vi "Creating Modulated Audio.vi"() -> ()   [LabVIEW 2019]
doc: "This application reads the selected audio file from its media storage. The audio is outputed through the Emona Communications Board for its modulation. After being modulated, the signal is inputed once again into the application. The modulated signal is now displayed through the Modulated Signal Graph."
uses:
  <vilib>/myRIO/Instrument Drivers/Onboard IO/AO Continuous/typedefs/AO Continuous Reference.ctl
  <vilib>/myRIO/Common/Instrument Driver Framework/Utilities/typedefs/myRIO Generic Hardware Reference.ctl
  <vilib>/myRIO/Common/Instrument Driver Framework/Utilities/typedefs/Hardware Version Enum.ctl
  <vilib>/myRIO/Common/Instrument Driver Framework/Utilities/typedefs/myRIO v1.0 Reference.ctl
  <vilib>/myRIO/Common/Instrument Driver Framework/Utilities/typedefs/Generic FPGA Reference.ctl
  <vilib>/myRIO/Common/Instrument Driver Framework/ELVIS III v1.0/AO Continuous/typedefs/AO Continuous Channels List.ctl
  <vilib>/myRIO/Common/Instrument Driver Framework/ELVIS III v1.0/AO Continuous/typedefs/ELVIS III v1.0 AO Continuous Channels Enum.ctl
  <vilib>/myRIO/Common/Instrument Driver Framework/ELVIS III v1.0/AO Continuous/typedefs/AO Continuous Channel Info.ctl
  <vilib>/userDefined/High Color/nirio_resource_hc.ctl
  <vilib>/myRIO/Instrument Drivers/Onboard IO/AO/typedefs/AO Reference.ctl
  <vilib>/myRIO/Common/Instrument Driver Framework/myRIO v1.0/AO/typedefs/AO Channels List.ctl
  <vilib>/myRIO/Common/Instrument Driver Framework/myRIO v1.0/AO/typedefs/AO Channels Enum.ctl
  <vilib>/myRIO/Common/Instrument Driver Framework/Utilities/typedefs/Analog Scaling Constants List.ctl
  <vilib>/myRIO/Common/Instrument Driver Framework/Utilities/typedefs/Analog Scaling Constants.ctl
  <vilib>/myRIO/Instrument Drivers/Onboard IO/AI Block/typedefs/AI Block Reference.ctl
  <vilib>/myRIO/Common/Instrument Driver Framework/myRIO v1.0/AI Block/typedefs/AI Block Channels List.ctl
  <vilib>/myRIO/Common/Instrument Driver Framework/myRIO v1.0/AI Block/typedefs/AI Block Channels Enum.ctl
  <vilib>/myRIO/Common/Instrument Driver Framework/ELVIS III v1.0/AO Continuous/vis/ELVIS III v1.1 Open AO (Continuous).vi
  <vilib>/myRIO/Common/Instrument Driver Framework/ELVIS III v1.0/AO/vis/ELVIS III v1.1 Open AO.vi
  <vilib>/myRIO/Common/Instrument Driver Framework/ELVIS III v1.0/AI Block/vis/ELVIS III v1.1 Open AI (N Samples).vi
  <vilib>/myRIO/Common/Instrument Driver Framework/Utilities/vis/Validate Channels.vi
  <vilib>/myRIO/Common/Instrument Driver Framework/ELVIS III v1.0/AO Continuous/vis/ELVIS III v1.0 Reserve AO Continuous.vi
  <vilib>/myRIO/Common/Instrument Driver Framework/ELVIS III v1.0/AO/vis/ELVIS III v1.0 Reserve AO.vi
  <vilib>/myRIO/Common/Instrument Driver Framework/ELVIS III v1.0/Resource Manager/vis/ELVIS III v1.0 Check For Different Banks.vi
  <vilib>/myRIO/Common/Instrument Driver Framework/ELVIS III v1.0/AI Block/vis/ELVIS III v1.0 AI Block Read.vi
  <vilib>/myRIO/Common/Instrument Driver Framework/ELVIS III v1.0/AO Continuous/vis/ELVIS III v1.1 Close AO Continuous.vi
  <vilib>/myRIO/Common/Instrument Driver Framework/ELVIS III v1.0/AO/vis/ELVIS III v1.0 Close AO.vi
  <vilib>/myRIO/Common/Instrument Driver Framework/ELVIS III v1.0/AI Block/vis/ELVIS III v1.0 Close AI Block.vi
  <vilib>/myRIO/Common/Instrument Driver Framework/myRIO v1.0/UART/vis/myRIO v1.0 Close UART.vi
  <vilib>/myRIO/Common/Instrument Driver Framework/ELVIS III v1.0/AO Continuous/vis/ELVIS III v1.0 Build MUX Configuration AO Continuous.vi
  <vilib>/myRIO/Common/Instrument Driver Framework/ELVIS III v1.0/AO/vis/ELVIS III v1.0 Build MUX Configuration AO.vi
  <vilib>/myRIO/Common/Instrument Driver Framework/Utilities/vis/Sample Rate To Ticks.vi
  <vilib>/myRIO/Common/Instrument Driver Framework/ELVIS III v1.0/AO Continuous/vis/ELVIS III v1.0 Unreserve AO Continuous.vi
  <vilib>/myRIO/Common/Instrument Driver Framework/ELVIS III v1.0/AO/vis/ELVIS III v1.0 Unreserve AO.vi
  <vilib>/myRIO/Common/Instrument Driver Framework/ELVIS III v1.0/AI Block/vis/ELVIS III v1.0 Unreserve AI Block.vi
  <vilib>/myRIO/Common/Instrument Driver Framework/ELVIS III v1.0/AI Block/vis/ELVIS III v1.0 Build MUX Configuration AI Block.vi
  <vilib>/Utility/VariantDataType/GetNumericInfo.vi
  <vilib>/Utility/error.llb/Error Cluster From Error Code.vi
  <vilib>/myRIO/Common/Instrument Driver Framework/ELVIS III v1.0/ELVIS III v1.1 Open.vi
  <vilib>/myRIO/Common/Instrument Driver Framework/ELVIS III v1.0/Resource Manager/vis/ELVIS III v1.0 Coerce AI Scaling.vi
  <vilib>/myRIO/Common/Instrument Driver Framework/ELVIS III v1.0/AI Block/vis/ELVIS III v1.0 Reserve AI Block.vi
  <vilib>/myRIO/Common/Instrument Driver Framework/ELVIS III v1.0/Resource Manager/vis/ELVIS III v1.0 Configure DMAs.vi
  <vilib>/myRIO/Common/Instrument Driver Framework/myRIO v1.0/myRIO v1.0 Close.vi
  <vilib>/myRIO/Common/Instrument Driver Framework/ELVIS III v1.0/Resource Manager/vis/ELVIS III v1.0 Reserve Channel List.vi
  <vilib>/myRIO/Common/Instrument Driver Framework/ELVIS III v1.0/AO Continuous/vis/ELVIS III v1.1 Stop AO Continuous.vi
  <vilib>/myRIO/Common/Instrument Driver Framework/ELVIS III v1.0/AO Continuous/vis/ELVIS III v1.0 AO Continuous Write.vi
  <vilib>/myRIO/Common/Instrument Driver Framework/ELVIS III v1.0/AO/vis/ELVIS III v1.0 Write AO.vi
  <vilib>/myRIO/Common/Instrument Driver Framework/ELVIS III v1.0/AO Continuous/vis/ELVIS III v1.1 Start AO Continuous.vi
  <vilib>/myRIO/Common/Instrument Driver Framework/myRIO v1.0/Resource Manager/vis/myRIO v1.0 Block Write Configuration.vi
  <vilib>/myRIO/Common/Instrument Driver Framework/ELVIS III v1.0/AI Block/vis/ELVIS III v1.0 AI Block Read Bank A.vi
  <vilib>/myRIO/Common/Instrument Driver Framework/ELVIS III v1.0/AI Block/vis/ELVIS III v1.0 AI Block Read Bank B.vi
  <vilib>/myRIO/Common/Instrument Driver Framework/ELVIS III v1.0/Resource Manager/vis/ELVIS III v1.0 Unreserve Channel List.vi
  <vilib>/myRIO/Common/Instrument Driver Framework/Utilities/vis/FPGA Ref Manager.vi
  <vilib>/myRIO/Common/Instrument Driver Framework/ELVIS III v1.0/ELVIS III v1.0 Reset FPGA.vi
  <vilib>/myRIO/Common/Instrument Driver Framework/myRIO v1.0/IRQ/vis/myRIO v1.0 IRQ Info FGV.vi
  <vilib>/myRIO/Common/Instrument Driver Framework/myRIO v1.0/IRQ/vis/myRIO v1.0 Timer IRQ Info FGV.vi
  <vilib>/myRIO/Common/Instrument Driver Framework/myRIO v1.0/IRQ/vis/myRIO v1.0 ISR Agent.vi
  <vilib>/myRIO/Instrument Drivers/Utilities/vis/Reset Index.vi
  <vilib>/myRIO/Common/Instrument Driver Framework/myRIO v1.0/Resource Manager/vis/myRIO v1.0 Block Write Resource Manager.vi
  <vilib>/myRIO/Instrument Drivers/Onboard IO/AI Block/vis/myRIO AI N Samples Open.xnode
  <vilib>/myRIO/Instrument Drivers/Onboard IO/AO/vis/myRIO AO Open.xnode
  <vilib>/myRIO/Instrument Drivers/Onboard IO/AO Continuous/vis/myRIO AO Continuous Open.xnode
  <vilib>/myRIO/Instrument Drivers/Utilities/Utilities.lvlib
  <vilib>/myRIO/Instrument Drivers/Onboard IO/AI Block/AI Block.lvlib
  <vilib>/myRIO/Instrument Drivers/Onboard IO/AO/AO.lvlib
  <vilib>/myRIO/Instrument Drivers/Onboard IO/AO Continuous/AO Continuous.lvlib
panel:
  in  "Select Audio":u16(ring)
  out "Message":dbl[](graph) caption="Message History"
  in  "Offset":dbl=1.0
  out "Modulated Signal":dbl[](graph)
  out "error out":errorcluster
  in  "Stop":bool
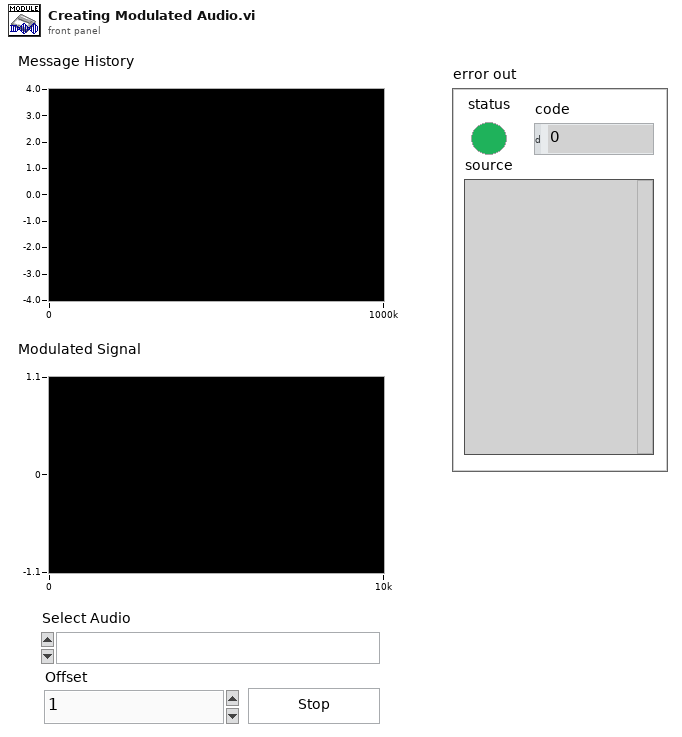
[diagram p1: front panel]
types:
  T1 = enum16{"open", "replace", "create", "open or create", "replace or create", "replace or create with confirmation"}
  T2 = typedef "nirio_resource_hc.ctl" = tag
  T3 = typedef "Hardware Version Enum.ctl" = enum16{"Unknown", "myRIO-1900", "myRIO-1950", "roboRIO", "NI ELVIS RIO CM", "ELVIS III"}
  T4 = typedef "AO Continuous.lvlib/AO Continuous Reference.ctl" = cluster{"myRIO Reference":T5, "AO (Continuous) Channels List":T8, "Channel Info":T10}
  T5 = typedef "myRIO Generic Hardware Reference.ctl" = cluster{"myRIO Model":T3, "myRIO Hardware Reference":T6}
  T6 = typedef "myRIO v1.0 Reference.ctl" = cluster{"Generic FPGA Reference":T7, "Allow multiple opens":bool}
  T7 = typedef "Generic FPGA Reference.ctl" = refnum<k20>
  T8 = typedef "AO Continuous Channels List.ctl" = T9[]
  T9 = typedef "ELVIS III v1.0 AO Continuous Channels Enum.ctl" = enum16{"Not Connected", "A/AO0 (Continuous)", "A/AO1 (Continuous)", "B/AO0 (Continuous)", "B/AO1 (Continuous)"}
  T10 = typedef "AO Continuous Channel Info.ctl" = cluster{"Channel Bitmask":u8[], "Channel Index":i32[], "Channel Number":u8}
  T11 = typedef "AO.lvlib/AO Reference.ctl" = cluster{"myRIO Reference":T5, "AO Channel List":T12, "AO Scaling Constant List":T14}
  T12 = typedef "AO Channels List.ctl" = T13[]
  T13 = typedef "AO Channels Enum.ctl" = enum16{"Not Connected", "AudioOut/Left", "AudioOut/Right", "C/AO0", "C/AO1", "A/AO0", "A/AO1", "B/AO0", "B/AO1"}
  T14 = typedef "Analog Scaling Constants List.ctl" = T15[]
  T15 = typedef "Analog Scaling Constants.ctl" = cluster{"LSB Weight (Volts)":dbl, "Offset (Volts)":dbl, "Signed?":bool}
  T16 = typedef "AI Block.lvlib/AI Block Reference.ctl" = cluster{"myRIO Reference":T5, "AI (N Samples) Channels List":T17, "AI (N Samples) Scaling Constants List":T15[]}
  T17 = typedef "AI Block Channels List.ctl" = T18[]
  T18 = typedef "AI Block Channels Enum.ctl" = enum16{"Not Connected", "A/AI0 (N Samples)", "A/AI1 (N Samples)", "A/AI2 (N Samples)", "A/AI3 (N Samples)", "A/AI4 (N Samples)", "A/AI5 (N Samples)", "A/AI6 (N Samples)", "A/AI7 (N Samples)", "A/AI0 (DIFF N Samples)", "A/AI1 (DIFF N Samples)", "A/AI2 (DIFF N Samples)", "A/AI3 (DIFF N Samples)", "B/AI0 (N Samples)", "B/AI1 (N Samples)", "B/AI2 (N Samples)", "B/AI3 (N Samples)", "B/AI4 (N Samples)", "B/AI5 (N Samples)", "B/AI6 (N Samples)", "B/AI7 (N Samples)", "B/AI0 (DIFF N Samples)", "B/AI1 (DIFF N Samples)", "B/AI2 (DIFF N Samples)", "B/AI3 (DIFF N Samples)"}
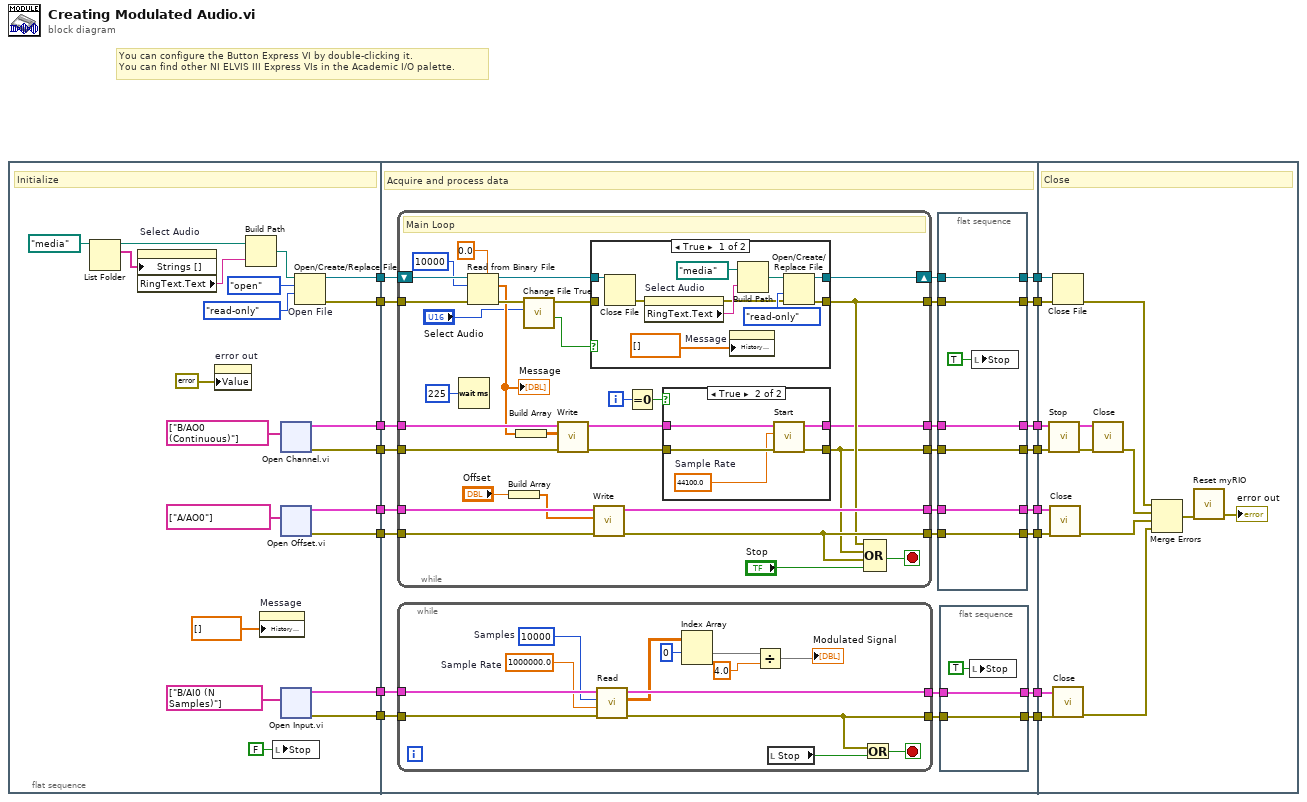
[diagram p0: block diagram]
diagram:
  # "You can configure the Button Express VI by double-clicking it.\nYou can find other NI ELVIS III Express VIs in the Academic I/O palette."
  n1 = flat-sequence {
    tunnel: [w36] -> w16
    tunnel: [w35] -> w15
    tunnel: [w33] -> w12
    tunnel: [w32] -> w11
    tunnel: [w27] -> w8
    tunnel: [w26] -> w7
    tunnel: [w23] -> w5
    tunnel: [w22] -> w4
    tunnel: w16 -> [w116]
    tunnel: w15 -> [w115]
    tunnel: [w93] -> w14
    tunnel: [w95] -> w13
    tunnel: w12 -> [w114]
    tunnel: w11 -> [w113]
    tunnel: [w99] -> w10
    tunnel: [w97] -> w9
    tunnel: w8 -> [w112]
    tunnel: w7 -> [w111]
    tunnel: [w105] -> w6
    tunnel: w5 -> [w110]
    tunnel: w4 -> [w109]
    tunnel: [w103] -> w3
    tunnel: [w101] -> w2
    tunnel: [w108] -> w1
    tunnel: w14 -> [w204]
    tunnel: w13 -> [w203]
    tunnel: w10 -> [w199]
    tunnel: w9 -> [w198]
    tunnel: w6 -> [w195]
    tunnel: w3 -> [w191]
    tunnel: w2 -> [w190]
    tunnel: w1 -> [w196]
    frame #0 {
      # "Initialize"
      n2 = List Folder(path=path "/media") -> (path out=w19:path, filenames=w20:string[])  [unwired: 3 in, 2 out]
      n3 = property on="Select Audio" class="Ring (strict)"("Strings []"=w20) -> ("RingText.Text"=w18:string)  [unwired: 2 in, 2 out]
      n4 = property on="error out" class="Clust (strict)"("Value"=errorcluster {"status"=FALSE, "code"=0, "source"=""} ("error constant")) -> ()  [unwired: 2 in, 2 out]
      n5 = Build Path(base path=w19, name or relative path=w18) -> (appended path=w28:path)
      n6 = property on="Message" class="WFChart (strict)"("History Data"=dbl[] []) -> ()  [unwired: 2 in, 2 out]
      n7 = local write "Stop"(FALSE ("Stop")) -> ()
      n8 = xnode "Open Channel.vi"("Channel Names"=tag[] ["B/AO0 (Continuous)"]) -> ("error out"=w22:errorcluster, "AO (Continuous) Ref Out"=w23:T4)  [unwired: 1 in]
      n9 = xnode "Open Offset.vi"("Channel Names"=tag[] ["A/AO0"]) -> ("error out"=w32:errorcluster, "AO Ref Out"=w33:T11)  [unwired: 2 in]
      n10 = xnode "Open Input.vi"("Channel Names"=tag[] ["B/AI0 (N Samples)"]) -> ("error out"=w36:errorcluster, "AI (N Samples) Ref Out"=w35:T16)  [unwired: 4 in]
      n11 = Open/Create/Replace File "Open File"(file path (use dialog)=w28, operation (0:open)=T1."open", access (0:read/write)=enum16{"read/write", "read-only", "write-only"}."read-only") -> (refnum out=w27:refnum<file>, error out=w26:errorcluster)  [unwired: 3 in, 1 out]
    }
    frame #1 {
      # "Acquire and process data"
      n12 = while {
        tunnel: w114 -> [w169]
        tunnel: w113 -> [w168]
        tunnel: [w165] -> w100
        tunnel: [w164] -> w98
        tunnel: w111 -> [w162]
        tunnel: [w155] -> w106
        tunnel: w109 -> [w149]
        tunnel: [w147] -> w102
        tunnel: w110 -> [w150]
        tunnel: [w148] -> w104
        shift-right: [w158] -> w107
        shift-left: w112 -> [w163]
        i -> [w151]
        stop <- w166 stop-if-true
        # "Main Loop"
        n13 = Wait (ms)(milliseconds to wait=u32 225) -> ()  [unwired: 1 out]
        n14 = Read from Binary File(5:0.0, 8:w162, 10:10000, 11:w163) -> (0:w145:errorcluster, 2:w142:dbl[], 3:w159:refnum<file>)  [unwired: 2 in, 1 out]
        "Message" <- w142
        n15 = Build Array("Offset") -> (w160:dbl[])
        n16 = Build Array(w142) -> (w146:dbl[][])
        n17 = call "Change File True.vi"("error in"=w145, "Numeric in"="Select Audio") -> ("error out"=w144:errorcluster, "Change song?"=w141:bool)  [unwired: 6 in, 1 out]
        n18 = call <vilib>:"Write.vi"("error in (no error)"=w149, "Data To Write"=w146, "AO (Continuous) Ref In"=w150) -> ("error out"=w153:errorcluster, "AO (Continuous) Ref Out"=w154:T4)  [unwired: 7 in]
        n19 = case shown="True" w141 {
          tunnel: [w183 w187] -> w155
          tunnel: w159 -> [w185 w188]
          tunnel: [w184 w188] -> w158
          tunnel: w144 -> [_ w187]
          frame True {
            n20 = Close File(refnum=w185) -> (error out=w178:errorcluster)  [unwired: 1 in, 1 out]
            n21 = property on="Select Audio" class="Ring (strict)"(error in=w178) -> (error out=w177:errorcluster, "RingText.Text"=w179:string)  [unwired: 1 in, 1 out]
            n22 = property on="Message" class="WFChart (strict)"("History Data"=dbl[] []) -> ()  [unwired: 2 in, 2 out]
            n23 = Build Path(base path=path "/media" ("path"), name or relative path=w179) -> (appended path=w181:path)
            n24 = Open/Create/Replace File ("Open File")(file path (use dialog)=w181, error in=w177, access (0:read/write)=enum16{"read/write", "read-only", "write-only"}."read-only") -> (refnum out=w184:refnum<file>, error out=w183:errorcluster)  [unwired: 3 in, 1 out]
          }
          frame False {
          }
        }
        n25 = call <vilib>:"Write.vi"("error in (no error)"=w168, "Values"=w160, "AO Ref In"=w169) -> ("error out"=w164:errorcluster, "AO Ref Out"=w165:T11)  [unwired: 6 in]
        n26 = Equal To 0?(x=w151) -> (x = 0?=w152:bool)
        n27 = case shown="True" w152 {
          tunnel: w154 -> [w171 w176]
          tunnel: w153 -> [w170 w175]
          tunnel: [w171 w174] -> w148
          tunnel: [w170 w173] -> w147
          frame False {
          }
          frame True {
            w172 = 44100.0  # Sample Rate
            n28 = call <vilib>:"Start.vi"("error in (no error)"=w175, "Sample Rate"=w172, "AO (Continuous) Ref In"=w176) -> ("error out"=w173:errorcluster, "AO (Continuous) Ref Out"=w174:T4)  [unwired: 7 in]
          }
        }
        n29 = Compound Arithmetic op=OR(w155, w147, w164, "Stop") -> (w166:bool)
      }
      n30 = while {
        tunnel: w115 -> [w139]
        tunnel: [w134] -> w96
        tunnel: w116 -> [w138]
        tunnel: [w136] -> w94
        stop <- w137 stop-if-true
        w128 = u32 10000  # Samples
        w129 = 1000000.0  # Sample Rate
        n31 = call <vilib>:"Read.vi"("error in (no error)"=w138, "Sample Rate [Hz]"=w129, "Number of Samples"=w128, "AI (N Samples) Ref In"=w139) -> ("error out"=w136:errorcluster, "Values"=w133:dbl[][], "AI (N Samples) Ref Out"=w134:T16)  [unwired: 5 in]
        n32 = Index Array(array=w133, index (row)=0) -> (element=w131:dbl[])  [unwired: 1 in]
        n33 = Divide(x=w131, y=4.0) -> (x/y=→"Modulated Signal":dbl[])
        n34 = local read "Stop"() -> (w135:bool)
        n35 = Or(x=w136, y=w135) -> (x .or. y?=w137:bool)
      }
      n36 = flat-sequence {
        tunnel: [w126] -> w108
        tunnel: w107 -> [w126]
        tunnel: w106 -> [w125]
        tunnel: [w125] -> w105
        tunnel: w104 -> [w124]
        tunnel: [w124] -> w103
        tunnel: w102 -> [w123]
        tunnel: [w123] -> w101
        tunnel: w100 -> [w122]
        tunnel: [w122] -> w99
        tunnel: w98 -> [w121]
        tunnel: [w121] -> w97
        frame #0 {
          n37 = local write "Stop"(TRUE ("Stop")) -> ()
        }
      }
      n38 = flat-sequence {
        tunnel: w96 -> [w119]
        tunnel: [w119] -> w95
        tunnel: w94 -> [w118]
        tunnel: [w118] -> w93
        frame #0 {
          n39 = local write "Stop"(TRUE ("Stop")) -> ()
        }
      }
    }
    frame #2 {
      # "Close"
      n40 = call <vilib>:"Stop.vi"("error in (no error)"=w190, "AO (Continuous) Ref In"=w191) -> ("error out"=w192:errorcluster, "AO (Continuous) Ref Out"=w193:T4)  [unwired: 8 in]
      n41 = call <vilib>:"Close.vi"("error in (no error)"=w198, "AO Ref In"=w199) -> ("error out"=w197:errorcluster)  [unwired: 9 in]
      n42 = Close File(refnum=w196, error in=w195) -> (error out=w194:errorcluster)  [unwired: 1 out]
      n43 = call <vilib>:"Close.vi"("error in (no error)"=w204, "AI (N Samples) Ref In"=w203) -> ("error out"=w202:errorcluster)  [unwired: 9 in]
      n44 = call <vilib>:"Close.vi"("error in (no error)"=w192, "AO (Continuous) Ref In"=w193) -> ("error out"=w189:errorcluster)  [unwired: 9 in]
      n45 = Merge Errors(w194, w189, w197, w202) -> (w200:errorcluster)
      n46 = call <vilib>:"Reset myRIO.vi"("error in (no error)"=w200) -> ("error out"=→"error out":errorcluster)  [unwired: 10 in]
    }
  }
